vi "ERIO WIN Batch Update SystemLink Tags.vi"(8 "error in (no error)":errorcluster, 9 "Tag Values":variant[](array[variant]), 10 "Tag Names":string[](array[string]), 11 "EEISysLink in":refnum<class "EEISysLink.lvclass">) -> (0 "error out":errorcluster, 3 "EEISysLink out":refnum<class "EEISysLink.lvclass">)   [LabVIEW 2016]
uses:
  EEI.LVLib/Class EEISysLink/EEISysLink.lvclass
  EEI.LVLib/Class EEISysLink/Controls/SL Tag Type.ctl
  EEI.LVLib/Class EEISysLink/Controls/SL Tag Scope.ctl
panel:
  # "NOTE: Tag names and values"
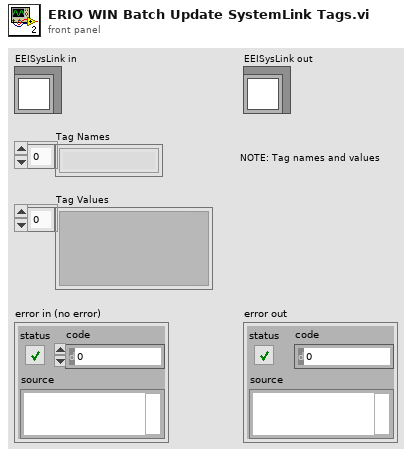
[diagram p1: front panel]
types:
  T1 = typedef "EEISysLink.lvclass/SL Tag Type.ctl" = enum16{"All", "Supervisor", "Worker"}
  T2 = typedef "EEISysLink.lvclass/SL Tag Scope.ctl" = enum16{"Local", "Server"}
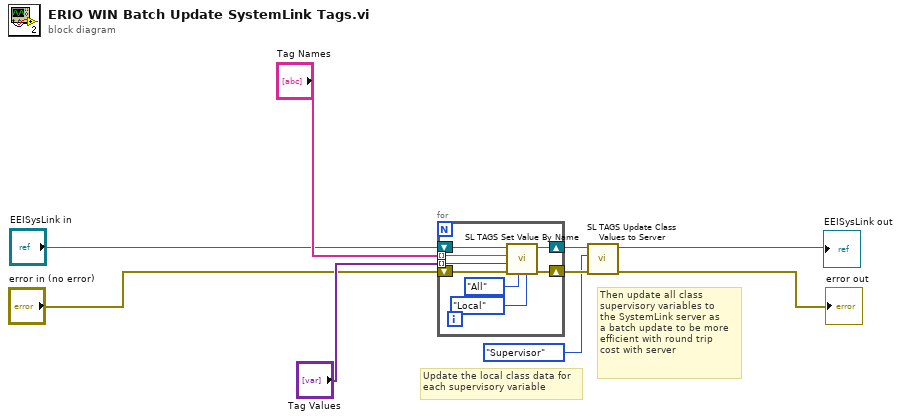
[diagram p0: block diagram]
diagram:
  # "Then update all class\nsupervisory variables to \nthe SystemLink server as\na batch update to be more\nefficient with round trip\ncost with server"
  # "Update the local class data for\neach supervisory variable"
  n1 = for {
    tunnel: "Tag Values" -> [w16] mode=indexing
    shift-right: [w11] -> w7
    shift-left: "error in (no error)" -> [w15]
    shift-right: [w12] -> w6
    shift-left: "EEISysLink in" -> [w17]
    tunnel: "Tag Names" -> [w10] mode=indexing
    n2 = call-dynamic "SL TAGS Set Value By Name.vi"("Tag Scope"=SL_Tag_Scope."Local", "Tag Type"=SL_Tag_Type."All", "error in (no error)"=w15, "Value"=w16, "Tag Name"=w10, "EEISysLink in"=w17) -> ("error out"=w11:errorcluster, "EEISysLink out"=w12:refnum<class "EEISysLink.lvclass">)  [unwired: 4 in]
  }
  n3 = call-dynamic "SL TAGS Update Class Values to Server.vi"("error in (no error)"=w7, "Tag Type"=SL_Tag_Type."Supervisor", "EEISysLink in"=w6) -> ("error out"=→"error out":errorcluster, "EEISysLink out"=→"EEISysLink out":refnum<class "EEISysLink.lvclass">)  [unwired: 7 in]
